vi "FineContrast_cleaned.vi"(0 "LightField Automation":refnum<class "LightField Automation.lvclass">, 1 "PZC200 Instrument Channel":string="GPIB/0:4,0", 2 "ExcWL_nm":dbl, 3 "PZC Error":errorcluster, 4 "Acq Time (ms) 2":dbl=500.0 caption="Acq Time :" min=0.0 max=360000.0 step=50.0, 5 "Acq Mode":T2=enum."Spectrum" caption="Mode :", 6 "CCD ROI":T4(ring), 7 "LightField Automation error":errorcluster, 8 "Shutter Device Reference":refnum<vi>, 9 "PZC Position Readout (usteps) 2":refnum<vi>, 10 "LinTFine Start":dbl, 11 "LinTFine End":dbl, 12 "Shutter Controls":refnum<vi>, 13 "Scan Spectrum Progess Bar 2":refnum<vi>, 14 "Stop Contrast 2":refnum<vi>, 15 "Pause Contrast 2":refnum<vi>, 16 "Contrast 1D Spectrum 2":refnum<vi>, 17 "LinTFine Step":dbl, 18 "Accumulations":dbl=1.0, 19 "Contrast Oscillations 2":refnum<vi>, 22 "Photodiode handle out":refnum<visa-resource-name> caption="instrument handle out", 23 "Photodiode error out":errorcluster caption="error out" {"code" format="%.0x"}) -> (20 "LightField Automation out":refnum<class "LightField Automation.lvclass">, 21 "PZC200 Instrument Channel 2":string, 24 "PZC Error 2":errorcluster, 25 "PZAPos & InstPow":dbl[][](array[numeric]), 26 "Spectra vs PZA":i32[][](array[numeric]), 27 "LightField Automation error  out":errorcluster)   [LabVIEW 2019]
uses:
  D:/Users/manip-thz/Documents/Controle_Manip_2020/Thorlabs.MotionControl.KCube.SolenoidCLI.dll
  Thorlabs.MotionControl.KCube.SolenoidCLI.dll
  Light Field/lightfield-automation-labview/LightField Automation.lvclass
  TypeDefs/AcqMode.ctl
panel:
  in  "Scan Translation Params":T1
  in  "Scan Translation Exp Params":T3
  out "InstPow":dbl[](array[numeric])
  out "ExcPow_uW":dbl
  out "WavelengthCalibration":dbl[](array[numeric])
  out "x+y":dbl
  out "PZA Positions":i32[](array[numeric])
  out "Contrast values":i32[](array[numeric])
  out "Contrast 1D Spectrum":cluster{dbl[], dbl[]}(graph) caption="64.0°"
  out "Contrast Oscillations":cluster{dbl[], dbl[]}(graph)
  in  "Pause Contrast":bool
  in  "Stop Contrast":bool
  out "PZC Position Readout (usteps)":dbl caption="Readout (usteps)" min=-8.0 max=392.0
  out "Scan Spectrum Progess Bar":u8(slide) scale=0.0..100.0
  out "KCube Shutter Device Reference":refnum<k24>
  out "Shutter Ctrls":u16(ring)
  # "ms"
types:
  T1 = cluster{"LinT Start Pos (mm)":dbl, "LinT Step Pos (mm)":dbl, "LinT End pos (mm)":dbl, "LinTFine Start Pos (usteps)":dbl, "LinTFines Step Pos (usteps)":dbl, "LinTFine End Pos (usteps)":dbl}
  T2 = typedef "AcqMode.ctl" = enum16{"Image", "Spectrum", "APD 1", "APD 2", "APD 1+2"}
  T3 = cluster{"Exposure Time (ms)":dbl, "Accumulations":dbl, "Excitation Wavelength (nm)":dbl, "Acq Mode":T2, "CCD ROI":enum16{"Custom ROI", "Full sensor", "Binned full sensor"}}
  T4 = enum16{"Custom ROI", "Full sensor", "Binned full sensor"}
  T5 = enum16{"Contrast", "Spectre", "Polarisation", "XY Intensity Map"}
  T6 = enum16{"Image", "Spectrum", "APD 1", "APD 2", "APD 1+2"}
  T7 = cluster{"Image":dbl[][][], "Frame Size":cluster{"F":i32, "Y":i32, "X":i32}}[]
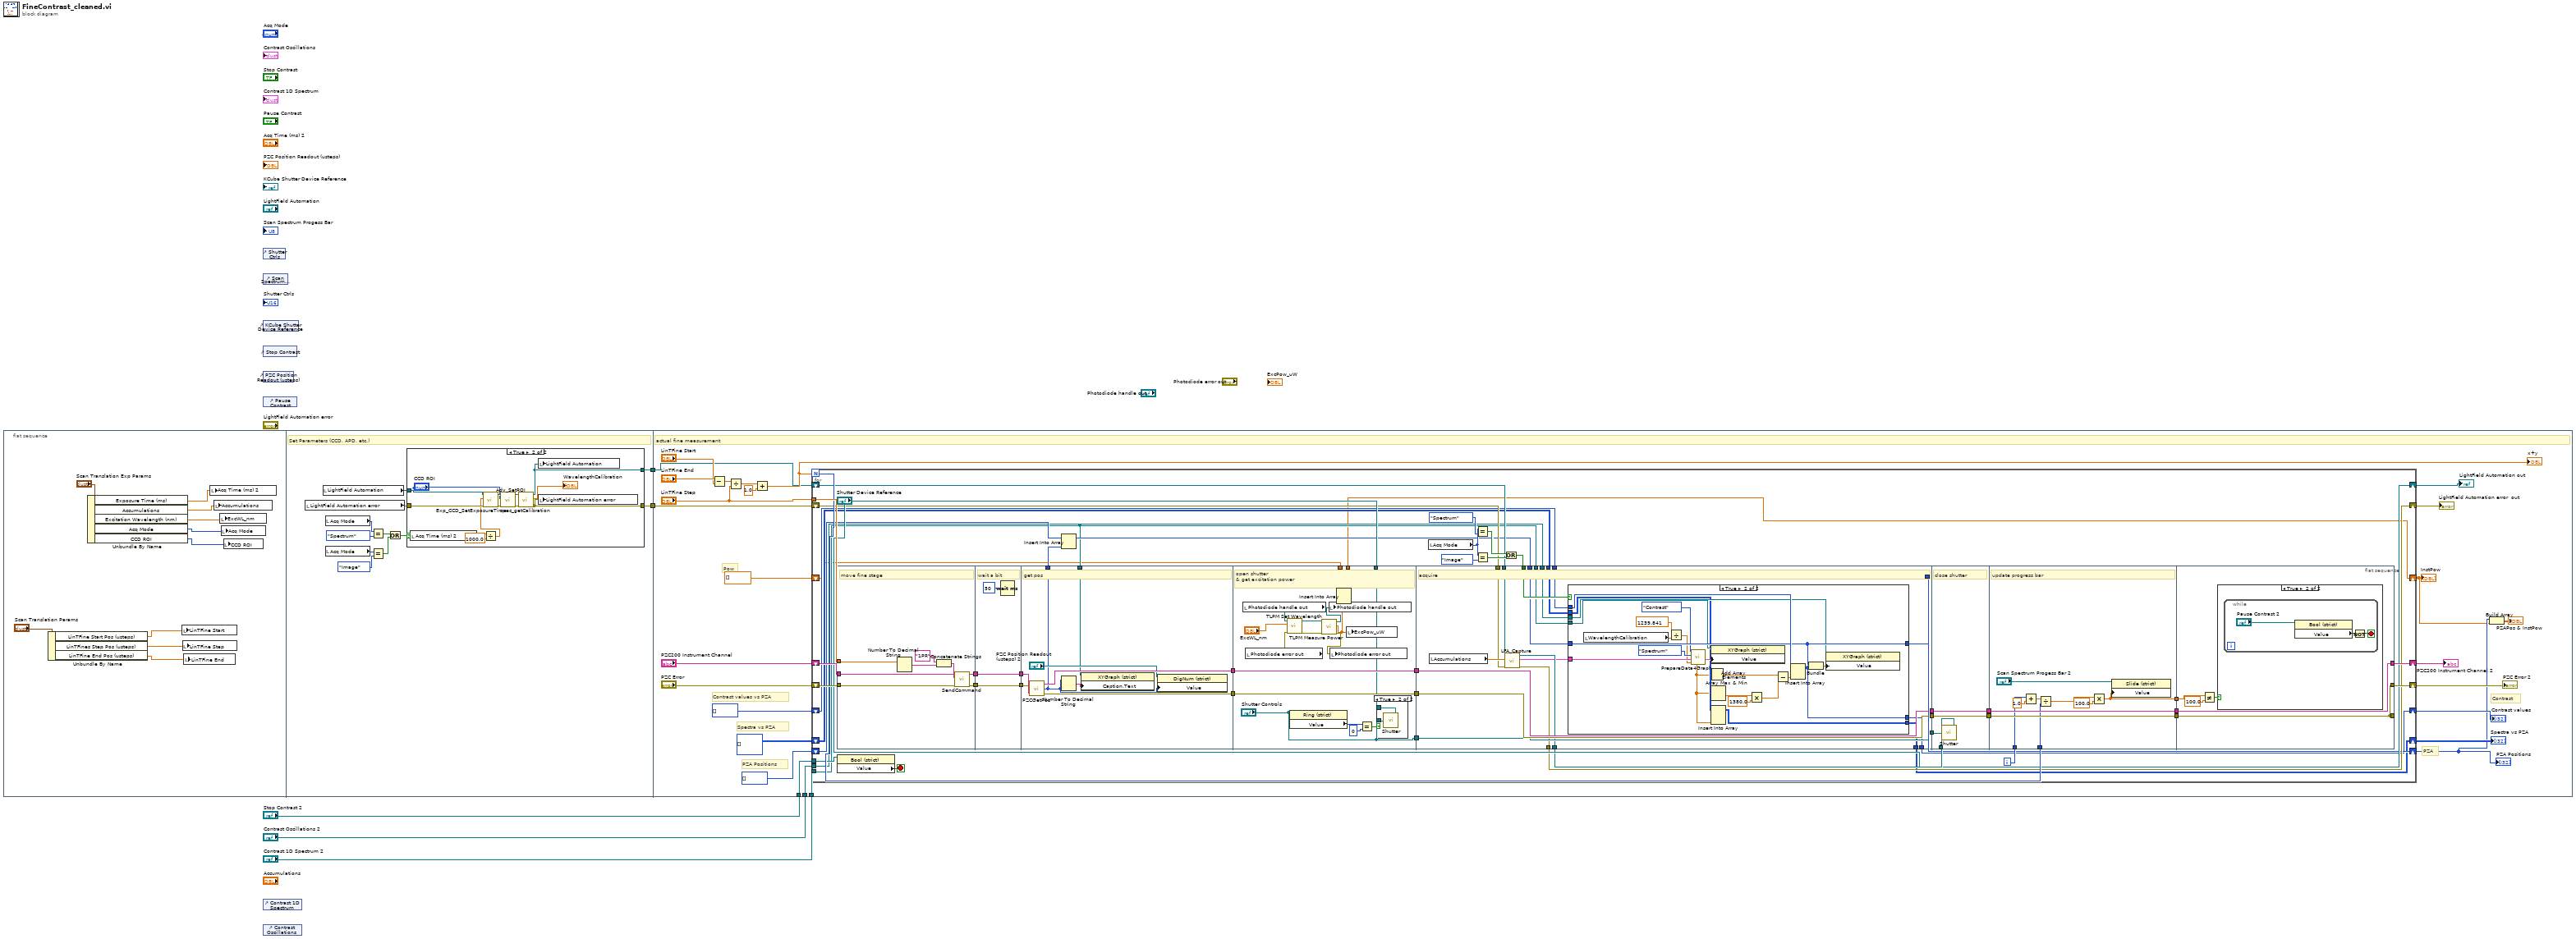
[diagram p0: block diagram]
diagram:
  n1 = flat-sequence {
    tunnel: [w19] -> w5
    tunnel: [w18] -> w4
    tunnel: w5 -> [w57]
    tunnel: w4 -> [w56]
    tunnel: "Stop Contrast 2" -> [w50]
    tunnel: "Contrast 1D Spectrum 2" -> [w49]
    tunnel: "Contrast Oscillations 2" -> [w48]
    frame #0 {
      n2 = Unbundle By Name("Scan Translation Params") -> ("LinTFine Start Pos (usteps)"=w8:dbl, "LinTFines Step Pos (usteps)"=w7:dbl, "LinTFine End Pos (usteps)"=w6:dbl)
      n3 = Unbundle By Name("Scan Translation Exp Params") -> ("Exposure Time (ms)"=w13:dbl, "Accumulations"=w12:dbl, "Excitation Wavelength (nm)"=w11:dbl, "Acq Mode"=w10:T2, "CCD ROI"=w9:T4)
      n4 = local write "LinTFine Start"(w8) -> ()
      n5 = local write "LinTFine Step"(w7) -> ()
      n6 = local write "LinTFine End"(w6) -> ()
      n7 = local write "Acq Time (ms) 2"(w13) -> ()
      n8 = local write "Accumulations"(w12) -> ()
      n9 = local write "ExcWL_nm"(w11) -> ()
      n10 = local write "Acq Mode"(w10) -> ()
      n11 = local write "CCD ROI"(w9) -> ()
    }
    frame #1 {
      # "Set Parameters (CCD, APD, etc.)"
      n12 = local read "LightField Automation error"() -> (w17:errorcluster)
      n13 = local read "LightField Automation"() -> (w16:refnum<class "LightField Automation.lvclass">)
      n14 = local read "Acq Mode"() -> (w26:T2)
      n15 = local read "Acq Mode"() -> (w22:T2)
      n16 = Equal?(x=w26, y=AcqMode."Spectrum" ("Acq Mode")) -> (x = y?=w24:bool)
      n17 = Equal?(x=w22, y=AcqMode."Image" ("Acq Mode")) -> (x = y?=w21:bool)
      n18 = Or(x=w24, y=w21) -> (x .or. y?=w20:bool)
      n19 = case shown="True" w20 {
        tunnel: [w28 w34] -> w19
        tunnel: [w27 w33] -> w18
        tunnel: w17 -> [w27 w38]
        tunnel: w16 -> [w28 w37]
        frame False {
        }
        frame True {
          n20 = local read "Acq Time (ms) 2"() -> (w31:dbl)
          n21 = Divide(x=w31, y=1000.0) -> (x/y=w29:dbl)
          n22 = call "Exp_CCD_SetExposureTime.vi"("error in (no error)"=w38, "Exposure Time (s)"=w29, "LightField Automation in"=w37) -> ("error out"=w40:errorcluster, "LightField Automation out"=w41:refnum<class "LightField Automation.lvclass">)  [unwired: 7 in]
          n23 = call "Adv_SetROI.vi"("error in (no error)"=w40, "ROI"="CCD ROI", "LightField Automation in"=w41) -> ("error out"=w35:errorcluster, "LightField Automation out"=w36:refnum<class "LightField Automation.lvclass">)  [unwired: 7 in]
          n24 = call "spec_getCalibration.vi"("error in (no error)"=w35, "LightField Automation in"=w36) -> ("error out"=w33:errorcluster, "ColumnCalibration"=→"WavelengthCalibration":dbl[], "LightField Automation out"=w34:refnum<class "LightField Automation.lvclass">)  [unwired: 7 in]
          n25 = local write "LightField Automation"(w34) -> ()
          n26 = local write "LightField Automation error"(w33) -> ()
        }
      }
    }
    frame #2 {
      # "Pow"
      # "Spectra vs PZA"
      # "Contrast"
      # "PZA"
      # "Contrast values vs PZA"
      # "PZA Positions"
      # "actual fine measurement"
      n27 = Subtract(x="LinTFine End", y="LinTFine Start") -> (x-y=w66:dbl)
      n28 = Divide(x=w66, y="LinTFine Step") -> (x/y=w65:dbl)
      n29 = Add(x=w65, y=1.0) -> (x+y=w63:dbl)
      "x+y" <- w63
      n30 = for {
        N: w63 -> [w101]
        tunnel: "LinTFine Step" -> [w117]
        shift-right: [w96] -> w59
        shift-left: "PZC200 Instrument Channel" -> [w115]
        shift-right: [w95] -> w58
        shift-left: "PZC Error" -> [w116]
        shift-right: [w84] -> w55
        shift-left: w57 -> [w86]
        shift-right: [w83] -> w54
        shift-left: w56 -> [w85]
        shift-right: [w73] -> w44
        shift-left: i32[] [] -> [w81]
        shift-right: [w72] -> w51
        shift-left: i32[] [] -> [w78]
        tunnel: w50 -> [w80]
        tunnel: w49 -> [w76]
        tunnel: w48 -> [w75]
        shift-right: [w71] -> w46
        shift-left: i32[][] [] -> [w74]
        shift-right: [w69] -> w43
        shift-left: dbl[] [] -> [w70]
        i -> [w102]
        stop <- w97 stop-if-true
        n31 = flat-sequence {
          tunnel: w117 -> [w125]
          tunnel: [w121] -> w114
          tunnel: [w120] -> w112
          tunnel: w116 -> [w119]
          tunnel: w115 -> [w118]
          tunnel: w114 -> [w128]
          tunnel: [w128] -> w113
          tunnel: w112 -> [w127]
          tunnel: [w127] -> w111
          tunnel: w113 -> [w136]
          tunnel: w111 -> [w135]
          tunnel: [w134] -> w110
          tunnel: [w133] -> w109
          tunnel: [w129] -> w82
          tunnel: w76 -> [w131]
          tunnel: w110 -> [w153]
          tunnel: w109 -> [w152]
          tunnel: "Shutter Device Reference" -> [w148]
          tunnel: [w153] -> w108
          tunnel: [w152] -> w107
          tunnel: ["Shutter Controls"] -> w93
          tunnel: w70 -> [w139]
          tunnel: [w137] -> w69
          tunnel: w108 -> [w173]
          tunnel: w107 -> [w172]
          tunnel: [w173] -> w106
          tunnel: [w172] -> w105
          tunnel: [w170] -> w94
          tunnel: w93 -> [w170]
          tunnel: w86 -> [w169]
          tunnel: w85 -> [w168]
          tunnel: [w167] -> w84
          tunnel: [w166] -> w83
          tunnel: w79 -> [w165]
          tunnel: w78 -> [w163]
          tunnel: w77 -> [w162]
          tunnel: w76 -> [w161]
          tunnel: w75 -> [w160]
          tunnel: w74 -> [w159]
          tunnel: [w158] -> w73
          tunnel: [w157] -> w72
          tunnel: [w156] -> w71
          tunnel: w106 -> [w201]
          tunnel: w105 -> [w200]
          tunnel: [w201] -> w104
          tunnel: [w200] -> w103
          tunnel: w94 -> [w199]
          tunnel: "Shutter Device Reference" -> [w198]
          tunnel: w104 -> [w211]
          tunnel: w103 -> [w210]
          tunnel: w102 -> [w204]
          tunnel: w101 -> [w203]
          tunnel: [w211] -> w100
          tunnel: [w210] -> w99
          tunnel: [w202] -> w98
          tunnel: [w212] -> _
          tunnel: [w216] -> w96
          tunnel: w100 -> [w216]
          tunnel: w99 -> [w212]
          tunnel: w98 -> [w214]
          tunnel: [w212] -> w95
          frame #0 {
            # "move fine stage"
            n32 = Number To Decimal String(number=w125) -> (decimal integer string=w123:string)  [unwired: 1 in]
            n33 = Concatenate Strings("1PR", w123) -> (w122:string)
            n34 = call "SendCommand.vi"("error in"=w119, "Command"=w122, "Instrument Channel"=w118) -> ("error out"=w120:errorcluster, "Instrument Channel out"=w121:string)  [unwired: 7 in]
          }
          frame #1 {
            # "wait a bit"
            n35 = Wait (ms)(milliseconds to wait=u32 50) -> ()  [unwired: 1 out]
          }
          frame #2 {
            # "get pos"
            n36 = call "PZCGetPos.vi"("error in"=w135, "Instrument Channel"=w136) -> ("Instrument Channel Out"=w134:string, "Position"=w129:i32, "error out"=w133:errorcluster)
            n37 = Number To Decimal String(number=w129) -> (decimal integer string=w130:string)  [unwired: 1 in]
            n38 = property class="XYGraph (strict)"(reference=w131, "Caption.Text"=w130) -> ()  [unwired: 1 in, 2 out]
            n39 = property class="DigNum (strict)"(reference="PZC Position Readout (usteps) 2", "Value"=w129) -> ()  [unwired: 1 in, 2 out]
          }
          frame #3 {
            # "open shutter\n& get excitation power"
            n40 = local read "Photodiode handle out"() -> (w143:refnum<visa-resource-name>)
            n41 = local read "Photodiode error out"() -> (w144:errorcluster)
            n42 = call <instrlib>:"TLPM Set Wavelength.vi"("error in (no error)"=w144, "Wavelength (0.0)"="ExcWL_nm", "instrument handle"=w143) -> ("error out"=w145:errorcluster, "instrument handle out"=w146:refnum<visa-resource-name>)  [unwired: 7 in]
            n43 = property class="Ring (strict)"(reference="Shutter Controls") -> ("Value"=w149:u16)  [unwired: 1 in, 2 out]
            n44 = call <instrlib>:"TLPM Measure Power.vi"("error in (no error)"=w145, "instrument handle"=w146) -> ("error out"=w140:errorcluster, "Power"=w138:dbl, "instrument handle out"=w141:refnum<visa-resource-name>)  [unwired: 7 in]
            n45 = local write "Photodiode handle out"(w141) -> ()
            n46 = local write "Photodiode error out"(w140) -> ()
            n47 = Insert Into Array(array=w139, new element=w138) -> (w137:dbl[])  [unwired: 1 in]
            n48 = local write "ExcPow_uW"(w138) -> ()
            n49 = Equal?(x=w149, y=u16 0) -> (x = y?=w150:bool)
            n50 = case shown="True" w150 {
              tunnel: "Shutter Controls" -> [_ w155]
              tunnel: w148 -> [_ w154]
              frame False {
              }
              frame True {
                n51 = call "Shutter.vi"("KCube Shutter Device Reference 2"=w154, "Shutter Ctrls 2"=w155) -> ()
              }
            }
          }
          frame #4 {
            # "acquire"
            n52 = local read "Accumulations"() -> (w171:dbl)
            n53 = call "LFA_Capture.vi"("error in (no error)"=w168, "Frames"=w171, "LightField Automation in"=w169) -> ("error out"=w166:errorcluster, "Data"=w164:T7, "LightField Automation out"=w167:refnum<class "LightField Automation.lvclass">)  [unwired: 6 in]
            n54 = case shown="True" w165 {
              tunnel: w164 -> [_ w197]
              tunnel: w163 -> [w175 w196]
              tunnel: w162 -> [w176 w194]
              tunnel: [w176 w194] -> w158
              tunnel: [w175 w193] -> w157
              tunnel: w161 -> [_ w192]
              tunnel: w160 -> [_ w191]
              tunnel: w159 -> [w174 w187]
              tunnel: [w174 w186] -> w156
              frame False {
              }
              frame True {
                n55 = local read "WavelengthCalibration"() -> (w179:dbl[])
                n56 = Divide(x=1239.841, y=w179) -> (x/y=w177:dbl[])
                n57 = call "PrepareData4Graph.vi"("Wavelength nm"=w177, "DataLF"=w197, "AcqMode"=T6."Spectrum", "Data type"=T5."Contrast") -> ("Spectrum"=w188:cluster{"Array 2":dbl[], "Array":dbl[]}, "PLInt out"=w182:dbl[])  [unwired: 2 in, 2 out]
                n58 = Add Array Elements(numeric array=w182) -> (sum=w185:dbl)
                n59 = property class="XYGraph (strict)"(reference=w192, "Value"=w188) -> ()  [unwired: 1 in, 2 out]
                n60 = Array Max & Min(array=w182) -> (min value=w181:dbl)  [unwired: 3 out]
                n61 = Insert Into Array(array=w187, new element=w182) -> (w186:i32[][])  [unwired: 2 in]
                n62 = Multiply(x=w181, y=1380.0) -> (x*y=w180:dbl)
                n63 = Subtract(x=w185, y=w180) -> (x-y=w184:dbl)
                n64 = Insert Into Array(array=w196, new element=w184) -> (w193:i32[])  [unwired: 1 in]
                n65 = Bundle(w194, w193) -> (w195:cluster{i32[], i32[]})  [unwired: 1 in]
                n66 = property class="XYGraph (strict)"(reference=w191, "Value"=w195) -> ()  [unwired: 1 in, 2 out]
              }
            }
          }
          frame #5 {
            # "close shutter"
            n67 = call "Shutter.vi"("KCube Shutter Device Reference 2"=w198, "Shutter Ctrls 2"=w199) -> ()
          }
          frame #6 {
            # "update progress bar"
            n68 = Add(x=w204, y=1.0) -> (x+y=w208:dbl)
            n69 = Divide(x=w208, y=w203) -> (x/y=w207:dbl)
            n70 = Multiply(x=w207, y=100.0) -> (x*y=w202:dbl)
            n71 = property class="Slide (strict)"(reference="Scan Spectrum Progess Bar 2", "Value"=w202) -> ()  [unwired: 1 in, 2 out]
          }
          frame #7 {
            n72 = Not Equal?(x=w214, y=100.0) -> (x != y?=w213:bool)
            n73 = case shown="True" w213 {
              frame False {
              }
              frame True {
                n74 = while {
                  stop <- w218 stop-if-true
                  n75 = property class="Bool (strict)"(reference="Pause Contrast 2") -> ("Value"=w219:bool)  [unwired: 1 in, 2 out]
                  n76 = Not(x=w219) -> (.not. x?=w218:bool)
                }
              }
            }
          }
        }
        n77 = property class="Bool (strict)"(reference=w80) -> ("Value"=w97:bool)  [unwired: 1 in, 2 out]
        n78 = Insert Into Array(array=w81, new element=w82) -> (w77:i32[])  [unwired: 1 in]
        n79 = local read "Acq Mode"() -> (w91:T2)
        n80 = Equal?(x=w91, y=AcqMode."Spectrum" ("Acq Mode")) -> (x = y?=w87:bool)
        n81 = Equal?(x=w91, y=AcqMode."Image" ("Acq Mode")) -> (x = y?=w88:bool)
        n82 = Or(x=w87, y=w88) -> (x .or. y?=w79:bool)
      }
      "LightField Automation out" <- w55
      "LightField Automation error  out" <- w54
      "Contrast values" <- w51
      "PZA Positions" <- w44
      "PZC Error 2" <- w58
      "PZC200 Instrument Channel 2" <- w59
      "Spectra vs PZA" <- w46
      "InstPow" <- w43
      n83 = Build Array(w44, w43) -> (→"PZAPos & InstPow":dbl[][])
    }
  }
  n84 = control-ref of="Shutter Ctrls"() -> ()  [unwired: 1 out]
  n85 = control-ref of="Scan Spectrum Progess Bar"() -> ()  [unwired: 1 out]
  n86 = control-ref of="KCube Shutter Device Reference"() -> ()  [unwired: 1 out]
  n87 = control-ref of="Stop Contrast"() -> ()  [unwired: 1 out]
  n88 = control-ref of="PZC Position Readout (usteps)"() -> ()  [unwired: 1 out]
  n89 = control-ref of="Pause Contrast"() -> ()  [unwired: 1 out]
  n90 = control-ref of="Contrast 1D Spectrum"() -> ()  [unwired: 1 out]
  n91 = control-ref of="Contrast Oscillations"() -> ()  [unwired: 1 out]
